vi "Initialize Attributes.vi"(8 "error in (no error)":errorcluster, 10 "Attribute Data":variant, 11 "PVConnection in":refnum<class "PVConnection.lvclass">) -> (0 "error out":errorcluster, 2 "Found?":bool, 3 "PVConnection out":refnum<class "PVConnection.lvclass">)   [LabVIEW 2016, in "CS++ProcessVariables.lvlib" / "PVConnection.lvclass"]
doc: "Initialize object attribute.\n\nUnique resources should be allocated elsewhere!"
uses:
  PVConnection.lvclass
  ProcessVariable/PV.lvclass
  ProcessVariable/PV.lvclass/PV.ctl
  PVConnection.lvclass/PVConnection.ctl
  <vilib>/Utility/error.llb/Error Cluster From Error Code.vi
  CS++BaseClasses/Base/CS++Base.lvclass
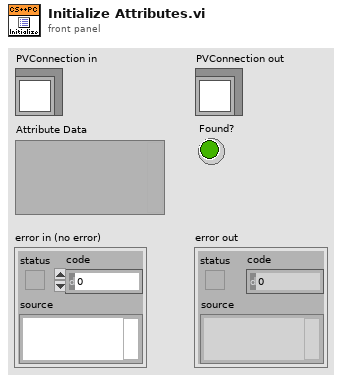
[diagram p1: front panel]
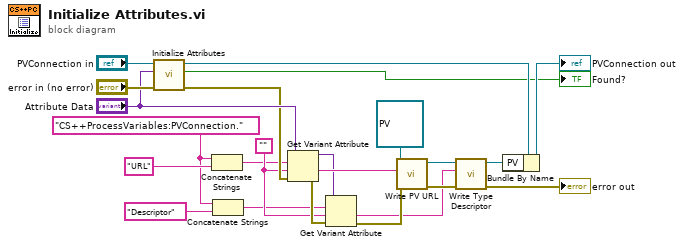
[diagram p0: block diagram]
diagram:
  w2 = "CS++ProcessVariables:PVConnection."
  w6 = ""
  n1 = call-parent "Initialize Attributes.vi"("error in (no error)"="error in (no error)", "Attribute Data"="Attribute Data", "CS++Base in"="PVConnection in") -> ("error out"=w19:errorcluster, "Found?"=→"Found?":bool, "CS++Base out"=w18:refnum<class "PVConnection.lvclass">)  [unwired: 6 in]
  n2 = Concatenate Strings(w2, "URL") -> (w4:string)
  n3 = Concatenate Strings(w2, "Descriptor") -> (w3:string)
  n4 = Get Variant Attribute(Variant="Attribute Data", name=w4, default value (empty Variant)=w6, error in=w19) -> (duplicate Variant=w8:variant, value=w15:string, error out=w10:errorcluster)  [unwired: 1 out]
  n5 = Get Variant Attribute(Variant=w8, name=w3, default value (empty Variant)=w6, error in=w10) -> (value=w5:string, error out=w9:errorcluster)  [unwired: 2 out]
  n6 = call "Write PV URL.vi"("error in (no error)"=w9, "PV URL"=w15, "PV in"=refnum<class "PV.lvclass"> refnum ("CS++ProcessVariables.lvlib:PV.lvclass")) -> ("error out"=w12:errorcluster, "PV out"=w14:refnum<class "PV.lvclass">)  [unwired: 7 in]
  n7 = call "Write Type Descriptor.vi"("error in (no error)"=w12, "Type Descriptor"=w5, "PV in"=w14) -> ("error out"=→"error out":errorcluster, "PV out"=w13:refnum<class "PV.lvclass">)  [unwired: 7 in]
  n8 = Bundle By Name(cluster=w18, "PV"=w13) -> (→"PVConnection out":refnum<class "PVConnection.lvclass">)
